vi "DAQ.Simulate Noisy AI.vi"(6 "Waveguide Cluster":T1={"I+"=0, "I-"=1, "V+"=2, "V-"=3, "Vsg"=4}, 8 "error in (no error)":errorcluster, 11 "Instrument.DAQ in":refnum<class "Instrument.DAQ.lvclass">) -> (0 "error out":errorcluster, 2 "Noisy Signal Graph":waveform(dbl)[](graph), 3 "Instrument.DAQ out":refnum<class "Instrument.DAQ.lvclass">, 4 "AI time (s)":dbl format="%#_6p")   [LabVIEW 2019, in "Instrument.Lockin.lvlib" / "Instrument.DAQ.lvclass"]
uses:
  Instrument.DAQ.lvclass
  Simulate/Waveguide Model--Cluster.ctl
  Instrument.DAQ.lvclass/Instrument.DAQ.ctl
panel:
  out "Signal Graph":waveform(dbl)[](graph)
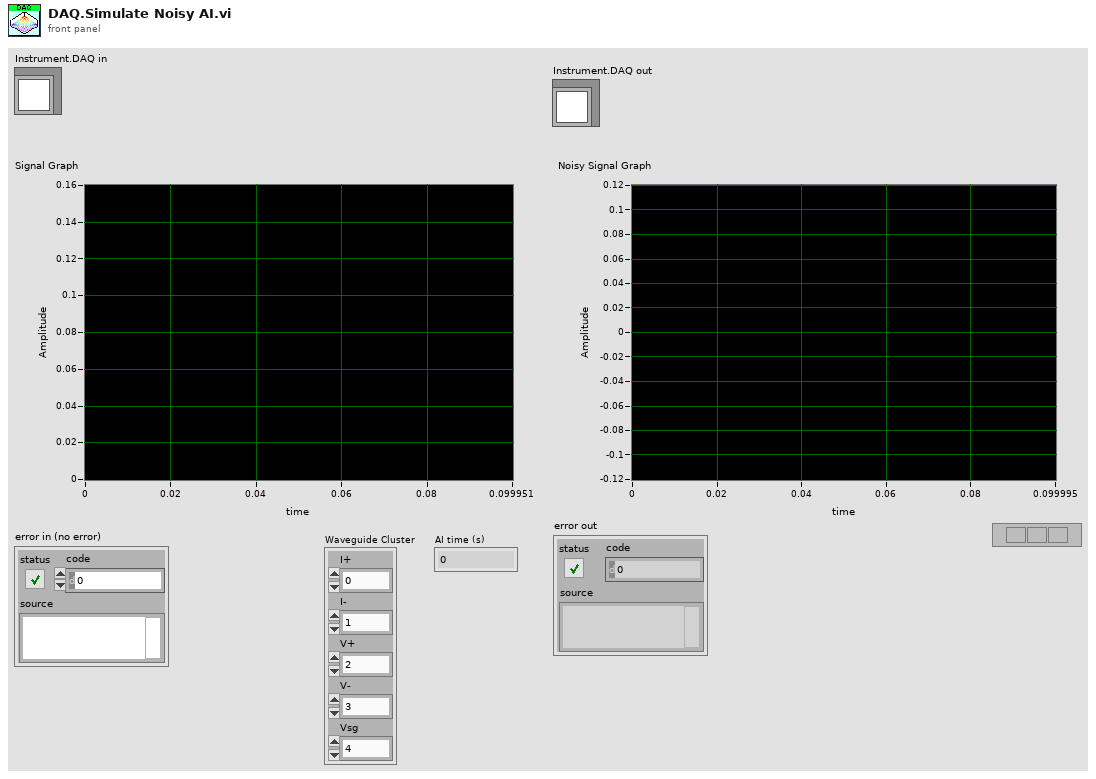
[diagram p1: front panel]
types:
  T1 = typedef "Instrument.Lockin.lvlib/Instrument.DAQ.lvclass/Waveguide Model--Cluster.ctl" = cluster{"I+":i32, "I-":i32, "V+":i32, "V-":i32, "Vsg":i32}
  T2 = typedef "Instrument.Lockin.lvlib/Instrument.DAQ.lvclass/DeviceInfo--Cluster.ctl" = cluster{"DeviceName":string, "DevIsSimulated":bool, "DeviceSerialNumber":string, "ProductType":string, "ProductCategory":i32, "ProductNumber":u32, "ChassisNumber":u32, "SlotNumber":u32, "ChassisName":string, "ChassisSerialNumber":string, "DevTemp":dbl, "SelfCal.LastDate/Time":string, "SelfCal.LastTemp":dbl, "calibration due?":bool}
  T3 = typedef "Instrument.Lockin.lvlib/Instrument.DAQ.lvclass/Simulation Mode--enum.ctl" = enum16{"AI = HW simulated", "AI = noise*AO", "AI = waveguide"}
  T4 = typedef "Instrument.Lockin.lvlib/Instrument.DAQ.lvclass/DAQ.Sampling.Sampling--Cluster.ctl" = cluster{"Fs":dbl, "#s":i32}
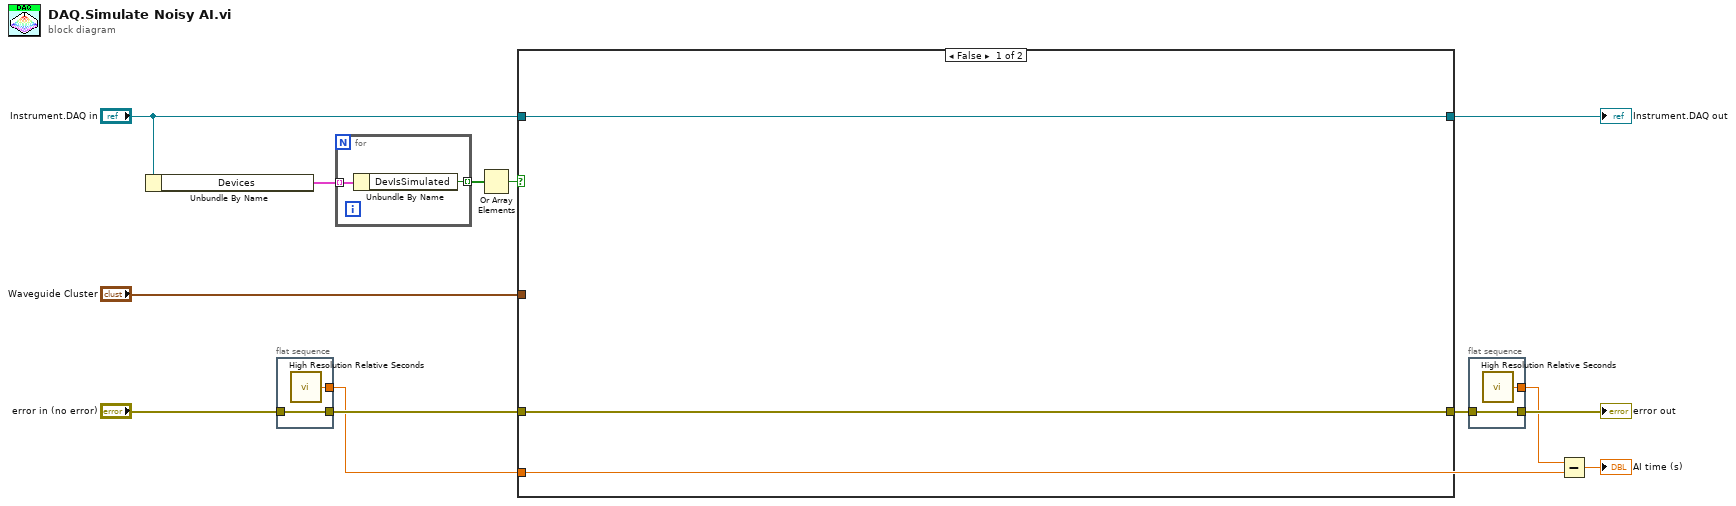
[diagram p0: block diagram]
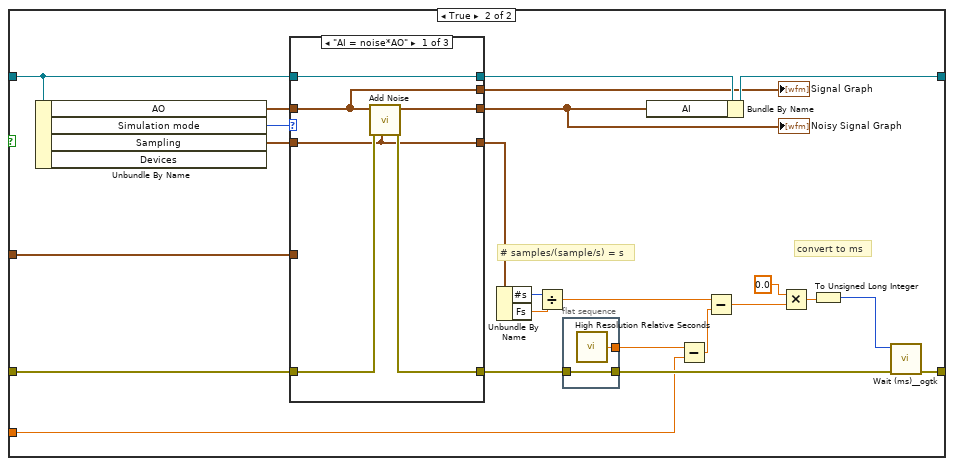
[diagram p2: hidden frame]
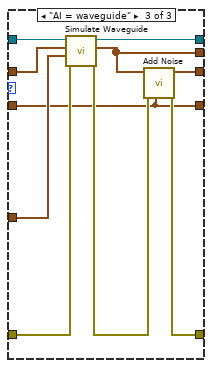
[diagram p4: hidden frame]
diagram:
  n1 = Unbundle By Name("Instrument.DAQ in") -> ("Devices"=w1:T2[])
  n2 = flat-sequence {
    tunnel: [w15] -> w9
    tunnel: "error in (no error)" -> [w15]
    tunnel: [w14] -> w5
    frame #0 {
      n3 = call <vilib>:"High Resolution Relative Seconds.vi"() -> ("relative seconds"=w14:dbl)
    }
  }
  n4 = for {
    tunnel: w1 -> [w17] mode=indexing
    tunnel: [w16] -> w3 mode=indexing
    n5 = Unbundle By Name(w17) -> ("DevIsSimulated"=w16:bool)
  }
  n6 = Or Array Elements(Boolean array=w3) -> (logical OR=w2:bool)
  n7 = case shown="False" w2 {
    tunnel: "Waveguide Cluster" -> [_ w40]
    tunnel: "Instrument.DAQ in" -> [w19 w23]
    tunnel: [w19 w38] -> w11
    tunnel: w9 -> [w18 w36]
    tunnel: [w18 w28] -> w8
    tunnel: w5 -> [_ w27]
    frame False {
    }
    frame True {
      # "convert to ms"
      # "# samples/(sample/s) = s"
      n8 = Unbundle By Name(w23) -> ("AO"=w22:waveform(dbl)[], "Simulation mode"=w21:T3, "Sampling"=w20:T4)  [unwired: 1 out]
      n9 = case shown="\"AI = noise*AO\"" w21 {
        tunnel: w36 -> [w48 w54 w62]
        tunnel: [w49 w54 w58] -> w39
        tunnel: [w50 w52 w60] -> w24
        tunnel: w40 -> [_ _ w61]
        tunnel: w22 -> [w46 w52 w65]
        tunnel: w23 -> [w51 w55 w64]
        tunnel: [w51 w55 w63] -> w37
        tunnel: w20 -> [w47 w53 w57]
        tunnel: [w47 w53 w57] -> w26
        tunnel: [w46 w52 w56] -> w25
        frame "AI = noise*AO" {
          n10 = call "Add Noise.vi"("Sampling"=w47, "error in (no error)"=w48, "AI []"=w46) -> ("error out"=w49:errorcluster, "AI + Noise"=w50:waveform(dbl)[])  [unwired: 7 in]
        }
        frame "AI = HW simulated" {
        }
        frame "AI = waveguide" {
          n11 = call "Simulate Waveguide.vi"("error in (no error)"=w62, "Waveguide Cluster"=w61, "AO"=w65, "Instrument.DAQ in"=w64) -> ("error out"=w59:errorcluster, "AI"=w56:waveform(dbl)[], "Instrument.DAQ out"=w63:refnum<class "Instrument.DAQ.lvclass">)  [unwired: 5 in]
          n12 = call "Add Noise.vi"("Sampling"=w57, "error in (no error)"=w59, "AI []"=w56) -> ("error out"=w58:errorcluster, "AI + Noise"=w60:waveform(dbl)[])  [unwired: 7 in]
        }
      }
      "Noisy Signal Graph" <- w24
      "Signal Graph" <- w25
      n13 = Unbundle By Name(w26) -> ("#s"=w41:i32, "Fs"=w42:dbl)
      n14 = Divide(x=w41, y=w42) -> (x/y=w33:dbl)
      n15 = flat-sequence {
        tunnel: [w45] -> w35
        tunnel: w39 -> [w45]
        tunnel: [w44] -> w34
        frame #0 {
          n16 = call <vilib>:"High Resolution Relative Seconds.vi"() -> ("relative seconds"=w44:dbl)
        }
      }
      n17 = Bundle By Name(cluster=w37, "AI"=w24) -> (w38:refnum<class "Instrument.DAQ.lvclass">)
      n18 = Subtract(x=w34, y=w27) -> (x-y=w43:dbl)
      n19 = Subtract(x=w33, y=w43) -> (x-y=w30:dbl)
      n20 = Multiply(x=0.0, y=w30) -> (x*y=w32:dbl)
      n21 = To Unsigned Long Integer(number=w32) -> (unsigned 32bit integer=w29:u32)
      n22 = call <userlib>:"Wait (ms)__ogtk.vi"("error in (no error)"=w35, "milliseconds to wait"=w29) -> ("error out"=w28:errorcluster)  [unwired: 8 in, 1 out]
    }
  }
  "Instrument.DAQ out" <- w11
  n23 = flat-sequence {
    tunnel: [w67] -> w7
    tunnel: w8 -> [w67]
    tunnel: [w66] -> w6
    frame #0 {
      n24 = call <vilib>:"High Resolution Relative Seconds.vi"() -> ("relative seconds"=w66:dbl)
    }
  }
  n25 = Subtract(x=w6, y=w5) -> (x-y=→"AI time (s)":dbl)
  "error out" <- w7
